vi "Pianoman.vi"() -> ()   [LabVIEW 2014]
uses:
  Color Sequence.ctl
  LED_Colors.ctl
  LED_Patterns.ctl
  Raw Sequence Cluster.ctl
  LED Message.ctl
panel:
  out "Raw Cluster":T1
  out "error out":errorcluster
  out "Current Color":T5={"Light Strip"={"Section 0"=0, "Section 1"=0, "Section 2"=0}, "Pattern"={"Pattern 0"=enum."Sweep", "Pattern 1"=enum."Sweep", "Pattern 2"=enum."Sweep"}, "Wait Time (ms)"=0}
  in  "Apply Button":bool
  in  "Sequence":T6
  in  "Stop Button":bool
  # "Copy this After array is ran\nto the primary program."
  # "Configuration Area"
  # "Demo Area"
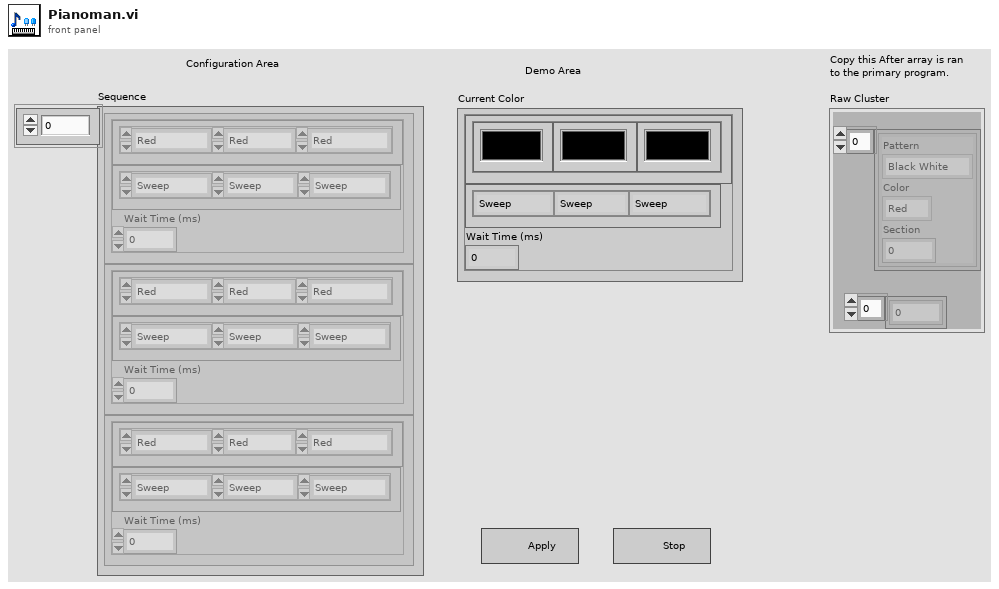
[diagram p1: front panel]
types:
  T1 = typedef "Raw Sequence Cluster.ctl" = cluster{"Pattern":T2[], "Timing":u32[]}
  T2 = typedef "LED Message.ctl" = cluster{"Pattern":T3, "Color":T4, "Section":u8}
  T3 = typedef "LED_Patterns.ctl" = enum8{"Black White", "Solid", "Blink", "Sweep", "Sleep"}
  T4 = typedef "LED_Colors.ctl" = enum8{"Red", "Green", "Blue", "Cyan", "Magenta", "Yellow"}
  T5 = cluster{"Light Strip":cluster{"Section 0":u32, "Section 1":u32, "Section 2":u32}, "Pattern":cluster{"Pattern 0":T3, "Pattern 1":T3, "Pattern 2":T3}, "Wait Time (ms)":u32}
  T6 = typedef "Color Sequence.ctl" = cluster{"Light Strip":cluster{"Color 0":T4, "Color 1":T4, "Color 2":T4}, "Pattern":cluster{"Pattern 0":T3, "Pattern 1":T3, "Pattern 2":T3}, "Wait Time (ms)":u32}[]
  T7 = cluster{"Color 0":T4, "Color 1":T4, "Color 2":T4}
  T8 = cluster{"Pattern 0":T3, "Pattern 1":T3, "Pattern 2":T3}
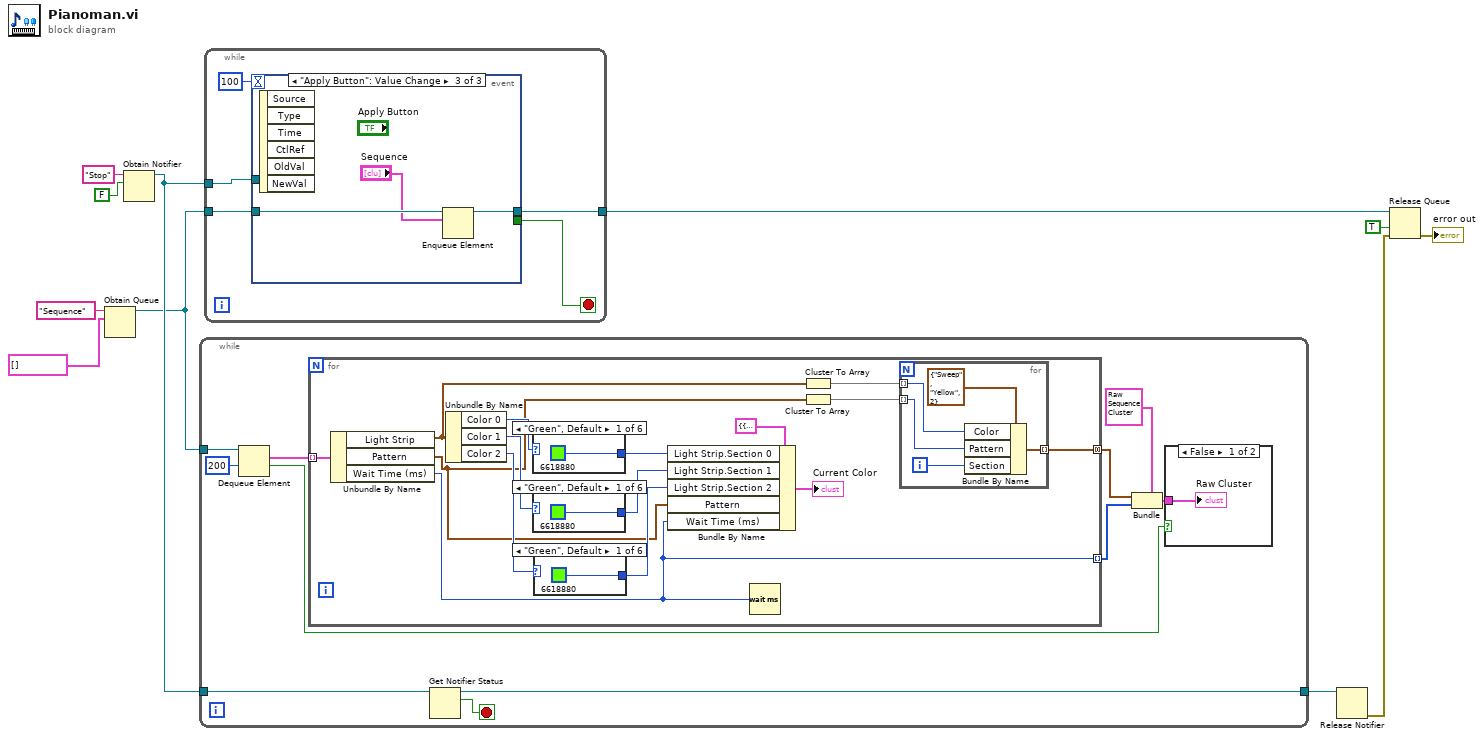
[diagram p0: block diagram]
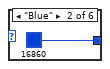
[diagram p3: hidden frame]
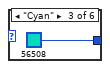
[diagram p4: hidden frame]
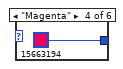
[diagram p5: hidden frame]
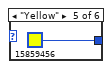
[diagram p6: hidden frame]
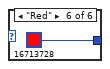
[diagram p7: hidden frame]
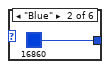
[diagram p8: hidden frame]
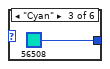
[diagram p9: hidden frame]
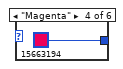
[diagram p10: hidden frame]
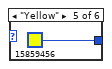
[diagram p11: hidden frame]
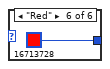
[diagram p12: hidden frame]
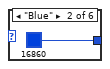
[diagram p13: hidden frame]
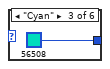
[diagram p14: hidden frame]
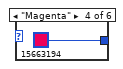
[diagram p15: hidden frame]
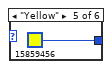
[diagram p16: hidden frame]
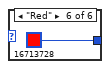
[diagram p17: hidden frame]
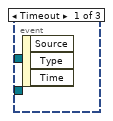
[diagram p18: hidden frame]
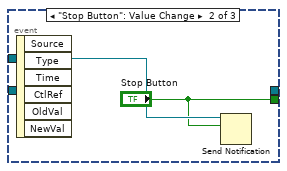
[diagram p19: hidden frame]
diagram:
  n1 = Obtain Queue(name (unnamed)="Sequence", element data type=T6 [] ("Sequence")) -> (queue out=w4:refnum<queue>)  [unwired: 3 in, 2 out]
  n2 = Obtain Notifier(name (unnamed)="Stop", notification data type=FALSE) -> (notifier out=w9:refnum<notifier>)  [unwired: 2 in, 2 out]
  n3 = while {
    tunnel: w9 -> [w21]
    tunnel: [w20] -> w8
    tunnel: w4 -> [w19]
    stop <- w22 stop-if-true
    n4 = Dequeue Element(queue=w19, timeout in ms (-1)=200) -> (element=w18:T6, timed out?=w14:bool)  [unwired: 1 in, 2 out]
    n5 = for {
      tunnel: w18 -> [w38] mode=indexing
      tunnel: [w25] -> w17 mode=concatenating
      tunnel: [w24] -> w16 mode=indexing
      n6 = Unbundle By Name(w38) -> ("Light Strip"=w29:T7, "Pattern"=w27:T8, "Wait Time (ms)"=w24:u32)
      n7 = Unbundle By Name(w29) -> ("Color 0"=w37:T4, "Color 1"=w36:T4, "Color 2"=w35:T4)
      n8 = case shown="\"Green\", Default" w37 {
        tunnel: [u32 6618880 u32 16860 u32 56508 u32 15663194 u32 15859456 u32 16713728] -> w33
        frame "Green", Default {
        }
        frame "Blue" {
        }
        frame "Cyan" {
        }
        frame "Magenta" {
        }
        frame "Yellow" {
        }
        frame "Red" {
        }
      }
      n9 = case shown="\"Green\", Default" w36 {
        tunnel: [u32 6618880 u32 16860 u32 56508 u32 15663194 u32 15859456 u32 16713728] -> w32
        frame "Green", Default {
        }
        frame "Blue" {
        }
        frame "Cyan" {
        }
        frame "Magenta" {
        }
        frame "Yellow" {
        }
        frame "Red" {
        }
      }
      n10 = case shown="\"Green\", Default" w35 {
        tunnel: [u32 6618880 u32 16860 u32 56508 u32 15663194 u32 15859456 u32 16713728] -> w31
        frame "Green", Default {
        }
        frame "Blue" {
        }
        frame "Cyan" {
        }
        frame "Magenta" {
        }
        frame "Yellow" {
        }
        frame "Red" {
        }
      }
      n11 = Bundle By Name(cluster=T5 {"Light Strip"={"Section 0"=0, "Section 1"=0, "Section 2"=0}, "Pattern"={"Pattern 0"=enum."Sweep", "Pattern 1"=enum."Sweep", "Pattern 2"=enum."Sweep"}, "Wait Time (ms)"=0} ("Current Color"), "Light Strip.Section 0"=w33, "Light Strip.Section 1"=w32, "Light Strip.Section 2"=w31, "Pattern"=w27, "Wait Time (ms)"=w24) -> (→"Current Color":T5)
      n12 = Wait (ms)(milliseconds to wait=w24) -> ()  [unwired: 1 out]
      n13 = Cluster To Array(cluster=w29) -> (array=w28:T4[])
      n14 = Cluster To Array(cluster=w27) -> (array=w26:T3[])
      n15 = for {
        tunnel: w28 -> [w42] mode=indexing
        tunnel: w26 -> [w41] mode=indexing
        tunnel: [w39] -> w25 mode=indexing
        i -> [w40]
        n16 = Bundle By Name(cluster=T2 {"Pattern"=enum."Sweep", "Color"=enum."Yellow", "Section"=2} ("LED Message"), "Color"=w42, "Pattern"=w41, "Section"=w40) -> (w39:T2)
      }
    }
    n17 = Get Notifier Status(notifier=w21) -> (notifier out=w20:refnum<notifier>, current notification=w22:bool)  [unwired: 1 in, 3 out]
    n18 = Bundle(cluster=T1 {"Pattern"=[{"Pattern"=enum."Sweep", "Color"=enum."Red", "Section"=0}, {"Pattern"=enum."Sweep", "Color"=enum."Red", "Section"=1}, {"Pattern"=enum."Sweep", "Color"=enum."Red", "Section"=2}, {"Pattern"=enum."Blink", "Color"=enum."Green", "Section"=0}, {"Pattern"=enum."Solid", "Color"=enum."Cyan", "Section"=1}, {"Pattern"=enum."Solid", "Color"=enum."Cyan", "Section"=2}, {"Pattern"=enum."Sweep", "Color"=enum."Yellow", "Section"=0}, {"Pattern"=enum."Sweep", "Color"=enum."Yellow", "Section"=1}, {"Pattern"=enum."Sweep", "Color"=enum."Yellow", "Section"=2}], "Timing"=[2000, 5000, 1000]} ("Raw Cluster"), "Pattern"=w17, "Timing"=w16) -> (w15:T1)
    n19 = case shown="False" w14 {
      tunnel: w15 -> [w23 _]
      frame False {
        "Raw Cluster" <- w23
      }
      frame True {
      }
    }
  }
  n20 = while {
    tunnel: w9 -> [w64]
    tunnel: w4 -> [w63]
    tunnel: [w62] -> w5
    stop <- w66 stop-if-true
    n21 = event shown="[2] \"Apply Button\": Value Change" {
      selector: _ -> [_ _ _]
      dyn-events: _ -> [_ _ _]
      timeout: 100 -> [_ _ _]
      tunnel: [_ "Stop Button" _] -> w66
      tunnel: w64 -> [_ w68 _]
      tunnel: w63 -> [_ _ w71]
      tunnel: [_ _ w69] -> w62
      event Timeout {
        n22 = event-data() -> ()  [unwired: 1 in, 3 out]
      }
      event "Stop Button": Value Change {
        n23 = event-data() -> ()  [unwired: 1 in, 6 out]
        n24 = Send Notification(notification="Stop Button", notifier=w68) -> ()  [unwired: 1 in, 2 out]
      }
      event "Apply Button": Value Change {
        n25 = event-data() -> ()  [unwired: 1 in, 6 out]
        n26 = Enqueue Element(queue=w71, element="Sequence") -> (queue out=w69:refnum<queue>)  [unwired: 2 in, 2 out]
      }
    }
  }
  n27 = Release Notifier(notifier=w8) -> (error out=w1:errorcluster)  [unwired: 2 in, 2 out]
  n28 = Release Queue(queue=w5, force destroy? (F)=TRUE, error in (no error)=w1) -> (error out=→"error out":errorcluster)  [unwired: 2 out]
